vi "Saturation Subtract.vi"   [LabVIEW 2020]
doc: "LabVIEW no longer supports this VI.\n\nComputes the difference between the inputs with a configurable output width, overflow handling, and an optional overflow output terminal."
uses:
  <vilib>/rvi/Arithmetic/AddSubMult/XNode/nirviSatArithmetic.xnode
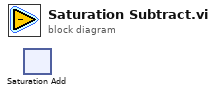
[diagram p0: block diagram]
diagram:
  n1 = xnode "Saturation Add"() -> ()  [unwired: 2 in, 1 out]
